vi "check_keithley-2400_is_connected.vi"(8 "error in (no error)":errorcluster, 11 "VISA resource name":refnum<visa-resource-name>="GPIB1::24::INSTR") -> (0 "error out":errorcluster)   [LabVIEW 2016]
uses:
  <instrlib>/Keithley 24XX/Keithley 24XX.lvlib
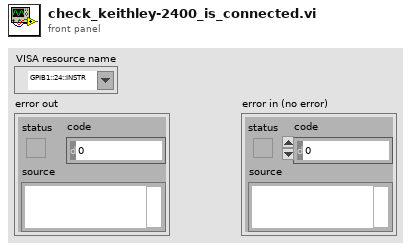
[diagram p1: front panel]
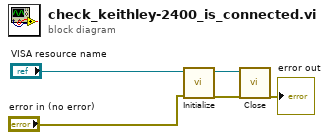
[diagram p0: block diagram]
diagram:
  n1 = call <instrlib>:"Initialize.vi"("error in (no error)"="error in (no error)", "VISA resource name"="VISA resource name") -> ("error out"=w3:errorcluster, "VISA resource name out"=w2:refnum<visa-resource-name>)  [unwired: 3 in, 5 out]
  n2 = call <instrlib>:"Close.vi"("error in (no error)"=w3, "VISA resource name"=w2) -> ("error out"=→"error out":errorcluster)  [unwired: 9 in]
